vi "New Triggered Subscription.vi"(7 "One-Shot? (T)":bool=TRUE, 8 "Trigger Value":variant, 9 "Trigger Condition":T1, 10 "Ignore Past Updates? (F)":bool, 11 "TriggeredSubscription In":refnum<class "TriggeredSubscription.lvclass">) -> (3 "TriggeredSubscription Out":refnum<class "TriggeredSubscription.lvclass">)   [LabVIEW 2017, in "SubscriptionPolicy.lvlib" / "TriggeredSubscription.lvclass"]
uses:
  TriggeredSubscription.lvclass
  Trigger Condition.ctl
  TriggeredSubscription.lvclass/TriggeredSubscription.ctl
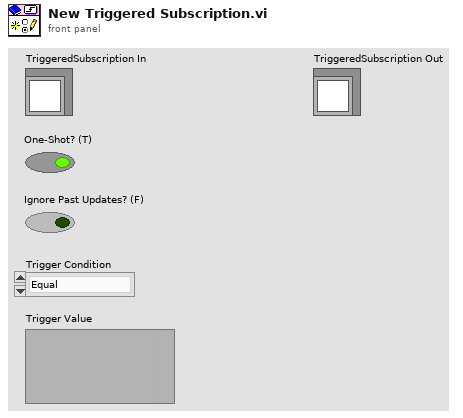
[diagram p1: front panel]
types:
  T1 = typedef "SubscriptionPolicy.lvlib/TriggeredSubscription.lvclass/Trigger Condition.ctl" = enum16{"Equal", "Not equal", "Greater than", "Less than", "Greater or equal", "Less or equal"}
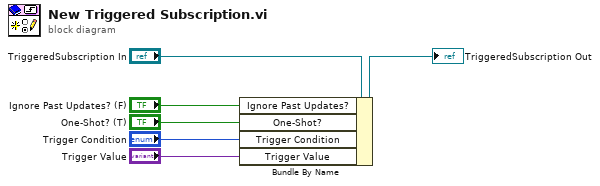
[diagram p0: block diagram]
diagram:
  n1 = Bundle By Name(cluster="TriggeredSubscription In", "Ignore Past Updates?"="Ignore Past Updates? (F)", "One-Shot?"="One-Shot? (T)", "Trigger Condition"="Trigger Condition", "Trigger Value"="Trigger Value") -> (→"TriggeredSubscription Out":refnum<class "TriggeredSubscription.lvclass">)
